vi "Extract subset.vi"() -> ()   [LabVIEW 2024]
panel:
  in  "File Path":path=path "\\\\myhome\\NHMFL/Projects/Pressure/Code/Alex/m005_092123.tdms"
  out "Waveform Graph":waveform(dbl)[](graph)
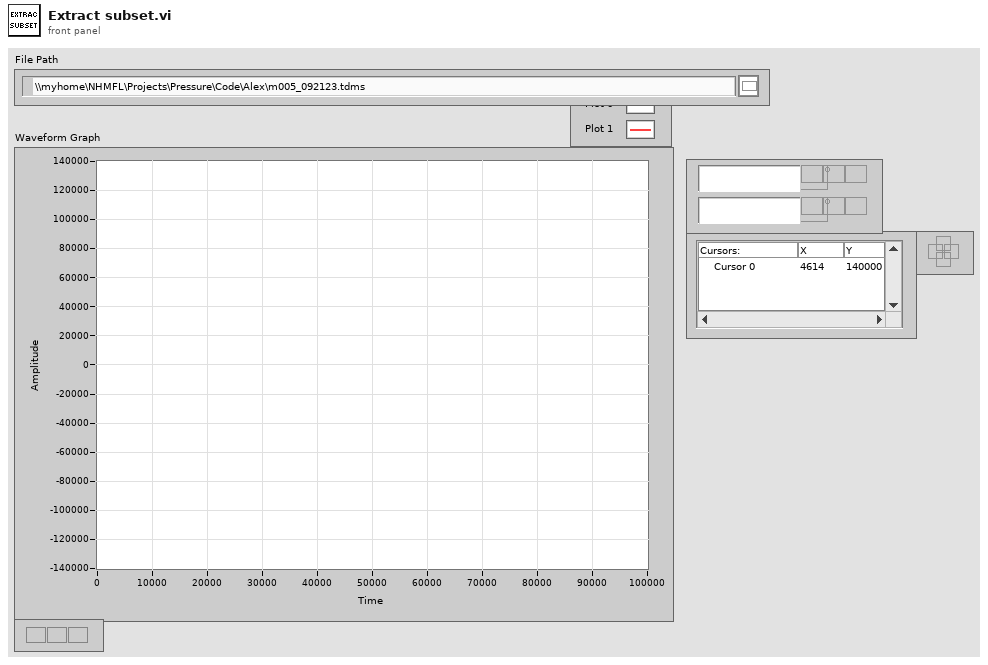
[diagram p1: front panel]
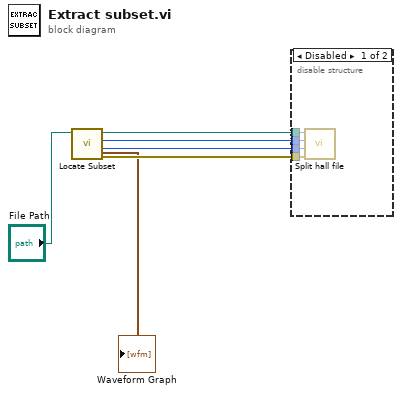
[diagram p0: block diagram]
diagram:
  n1 = call "Locate Subset.vi"("File Path"="File Path") -> ("error out"=w4:errorcluster, "Length out"=w5:i32, "Start Index out"=w6:i32, "file path out"=w3:path, "Waveform Graph"=→"Waveform Graph":waveform(dbl)[])  [unwired: 6 in]
  n2 = disable-structure shown="Disabled" {
    disable-tunnel: w6 -> [w10 _]
    disable-tunnel: w5 -> [w9 _]
    disable-tunnel: w4 -> [w8 _]
    disable-tunnel: w3 -> [w7 _]
    frame Disabled {
      n3 = call "Split hall file.vi"("error in"=w8, "Length"=w9, "Start Index"=w10, "File Path"=w7) -> ()  [unwired: 7 in, 1 out]
    }
    frame Enabled {
    }
  }
